vi "Forward_Kinematics_v1.vi"(1 "theta 3":dbl, 2 "theta 2":dbl, 3 "theta 1":dbl) -> (0 "position":dbl[](array[numeric]))   [LabVIEW 2010]
doc: "This VI takes in the theta 1(deg), theta 2(deg), and theta 3(mm) for L1, L2, and L3 of IRISS. The output will be a position array [px, py, pz]."
uses:
  <vilib>/Analysis/NI_AALBase.lvlib
  <vilib>/Analysis/baseanly.llb/Real A x B.vi
  <vilib>/Analysis/Matrix/Datatypes/RealMatrix.ctl
  <vilib>/Analysis/Matrix/NI_Matrix.lvlib
panel:
  out "T3 mtx":T1
  out "T2 mtx":T1
  out "T1 mtx":T1
  out "cos th2":dbl
  out "sin th2":dbl
  out "cos th1":dbl
  out "sin th1":dbl
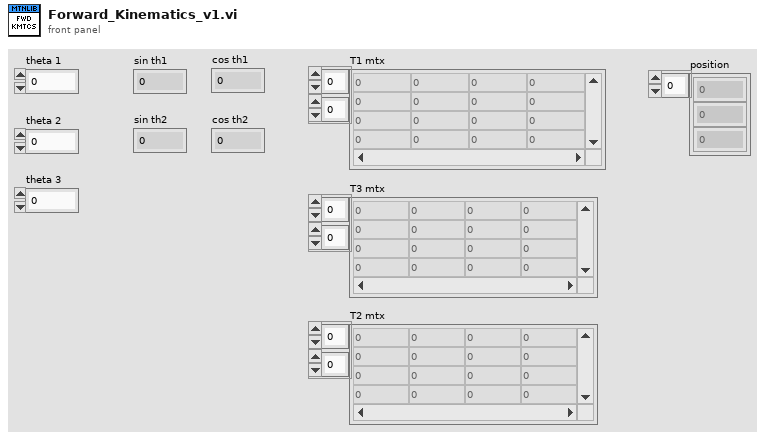
[diagram p1: front panel]
types:
  T1 = typedef "NI_Matrix.lvlib/RealMatrix.ctl" = dbl[][]
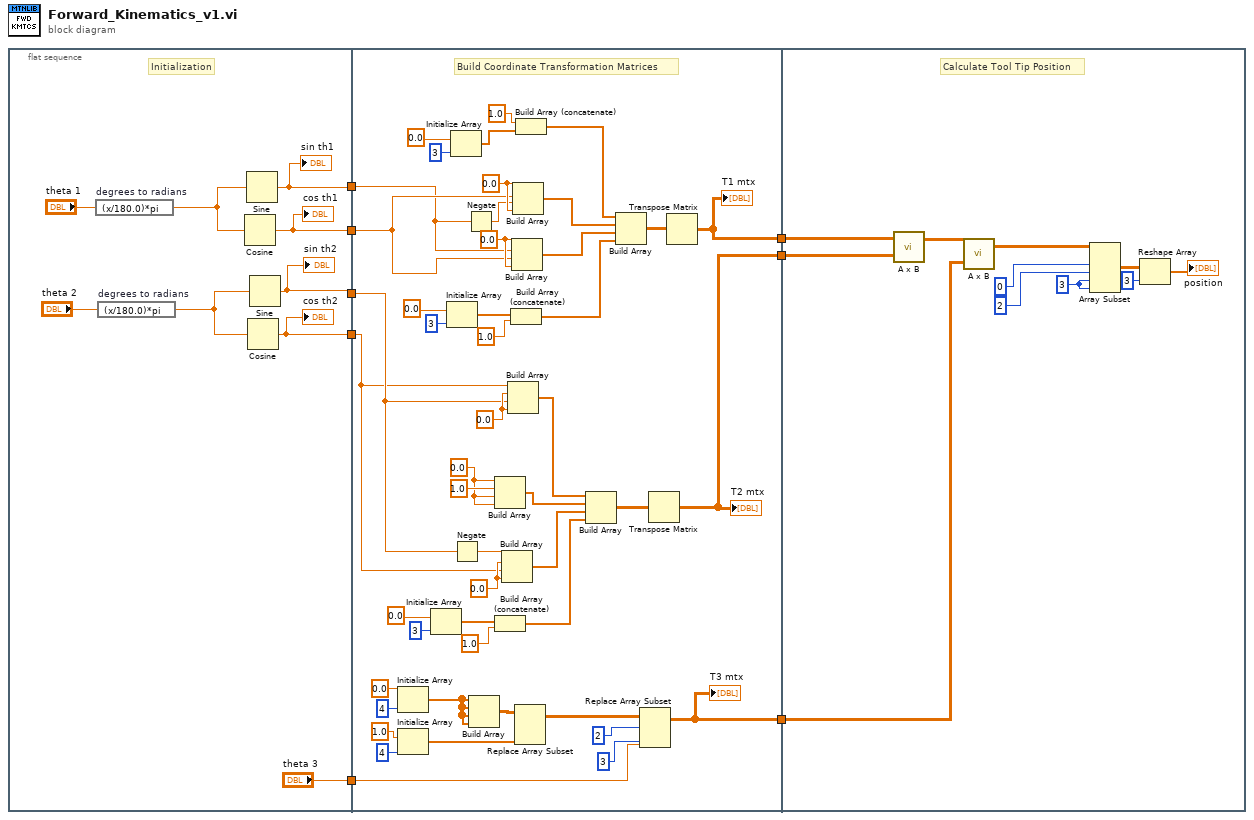
[diagram p0: block diagram]
diagram:
  n1 = flat-sequence {
    tunnel: [w13] -> w8
    tunnel: [w12] -> w7
    tunnel: [w11] -> w6
    tunnel: [w10] -> w5
    tunnel: ["theta 3"] -> w4
    tunnel: w8 -> [w25]
    tunnel: w7 -> [w24]
    tunnel: w6 -> [w22]
    tunnel: w5 -> [w23]
    tunnel: w4 -> [w21]
    tunnel: [w20] -> w3
    tunnel: [w19] -> w2
    tunnel: [w18] -> w1
    tunnel: w3 -> [w68]
    tunnel: w2 -> [w67]
    tunnel: w1 -> [w66]
    frame #0 {
      # "Initialization"
      n2 = expression code="(x/180.0)*pi" "degrees to radians"("theta 1") -> (w16:dbl)
      n3 = expression code="(x/180.0)*pi" "degrees to radians"("theta 2") -> (w14:dbl)
      n4 = Cosine(x=w16) -> (cos(x)=w13:dbl)
      "cos th1" <- w13
      n5 = Sine(x=w16) -> (sin(x)=w12:dbl)
      "sin th1" <- w12
      n6 = Cosine(x=w14) -> (cos(x)=w11:dbl)
      "cos th2" <- w11
      n7 = Sine(x=w14) -> (sin(x)=w10:dbl)
      "sin th2" <- w10
    }
    frame #1 {
      w46 = 0.0 ("element")
      w47 = 0.0 ("element")
      w40 = 0.0 ("element")
      w60 = 0.0 ("element")
      w61 = 0.0 ("element")
      # "Build Coordinate Transformation Matrices"
      n8 = Initialize Array(0.0 ("element"), 4 ("dimension size")) -> (w36:dbl[])
      n9 = Initialize Array(1.0 ("element"), 4 ("dimension size")) -> (w32:dbl[])
      n10 = Initialize Array(0.0 ("element"), 3 ("dimension size")) -> (w50:dbl[])
      n11 = Initialize Array(0.0 ("element"), 3 ("dimension size")) -> (w57:dbl[])
      n12 = Initialize Array(0.0 ("element"), 3 ("dimension size")) -> (w64:dbl[])
      n13 = Negate(x=w23) -> (-x=w45:dbl)
      n14 = Negate(x=w24) -> (-x=w28:dbl)
      n15 = Build Array(w36, w36, w36, w36) -> (w35:dbl[][])
      n16 = Build Array(w40, 1.0 ("element"), w40, w40) -> (w43:dbl[])
      n17 = Build Array (concatenate)(w50, 1.0 ("element")) -> (w39:dbl[])
      n18 = Build Array(w45, w46, w22, w46) -> (w42:dbl[])
      n19 = Build Array(w22, w47, w23, w47) -> (w44:dbl[])
      n20 = Build Array (concatenate)(w57, 1.0 ("element")) -> (w52:dbl[])
      n21 = Build Array(w60, w24, w25, w60) -> (w53:dbl[])
      n22 = Build Array(w61, w25, w28, w61) -> (w54:dbl[])
      n23 = Replace Array Subset(array=w35, new element=w32) -> (w31:T1)  [unwired: 2 in]
      n24 = Build Array (concatenate)(1.0 ("element"), w64) -> (w55:dbl[])
      n25 = Build Array(w44, w43, w42, w39) -> (w26:T1)
      n26 = Build Array(w55, w54, w53, w52) -> (w27:T1)
      n27 = Replace Array Subset(array=w31, new element=w21, index (row)=2 ("disabled index (row)"), index (col)=3 ("disabled index (col)")) -> (w18:T1)
      "T3 mtx" <- w18
      n28 = Transpose Matrix(1:w26) -> (0:w19:T1)
      "T2 mtx" <- w19
      n29 = Transpose Matrix(1:w27) -> (0:w20:T1)
      "T1 mtx" <- w20
    }
    frame #2 {
      w72 = 3 ("column 1")
      # "Calculate Tool Tip Position"
      n30 = call-poly <vilib>:"A x B.vi"("B"=w67, "A"=w68) -> ("A x B"=w76:T1)  [unwired: 1 out]
      n31 = call-poly <vilib>:"A x B.vi"("B"=w66, "A"=w76) -> ("A x B"=w75:T1)  [unwired: 1 out]
      n32 = Array Subset(array=w75, index (row)=0 ("row 1"), length (row)=2 ("row N"), index (col)=w72, length (col)=w72) -> (w71:T1)
      n33 = Reshape Array(w71, 3 ("dimension size")) -> (→"position":dbl[])
    }
  }
